vi "test windows positionierung.vi"() -> ()   [LabVIEW 2014, in "POLARIS Vision utility.lvlib"]
uses:
  POLARIS Vision utility.lvlib
panel:
  in  "Path":path
  in  "stop":bool
  in  "String 2":string
  out "String":string
  in  "Numeric":dbl
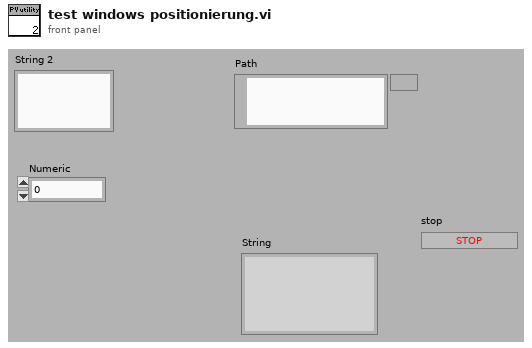
[diagram p1: front panel]
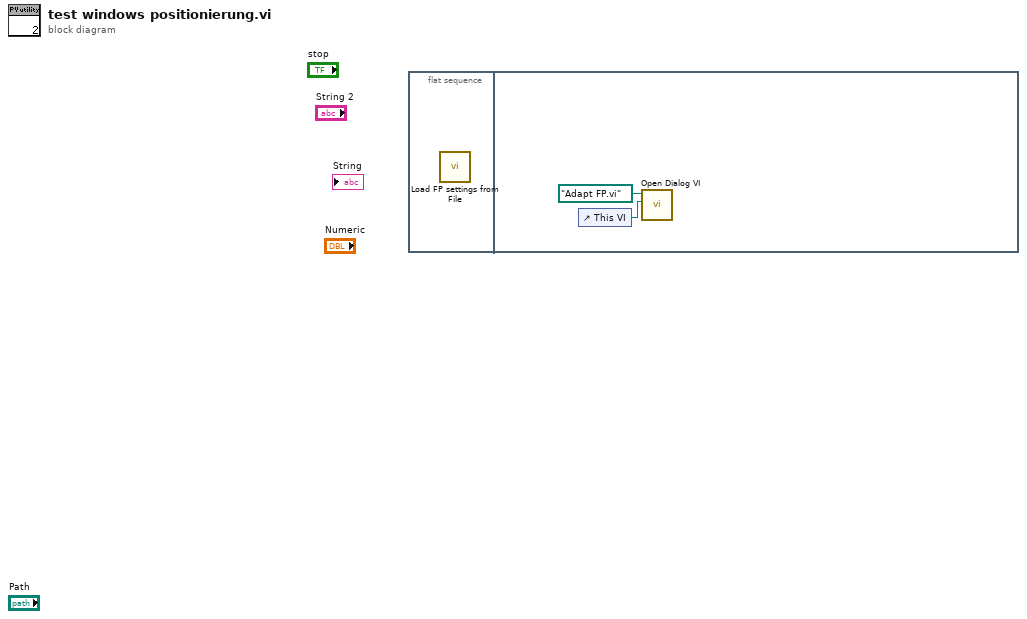
[diagram p0: block diagram]
diagram:
  n1 = flat-sequence {
    frame #0 {
      n2 = call "Load FP settings from File.vi"() -> ()  [unwired: 11 in, 1 out]
    }
    frame #1 {
      n3 = control-ref of="This VI"() -> (w2:refnum<vi>)
      n4 = call "Open Dialog VI.vi"("ref for signalling"=w2, "vi path"=path "Adapt FP.vi") -> ()  [unwired: 9 in, 1 out]
    }
  }
